vi "timekeeper locked (g).vi"() -> ()   [LabVIEW 2011, in "EPS_Timekeeper.lvlib"]
uses:
  <vilib>/addons/Electrical Power/Example Support/PMU/Time Keeper/EPS_Timekeeper.lvlib
panel:
  out "timekeeper locked (g)":bool
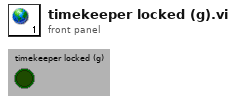
[diagram p1: front panel]
diagram:
